vi "INI_DS1104Z.vi"(11 "VISA resource name":refnum<visa-resource-name>) -> (3 "VISA resource name out":refnum<visa-resource-name>)   [LabVIEW 2018]
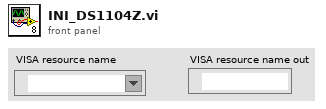
[diagram p1: front panel]
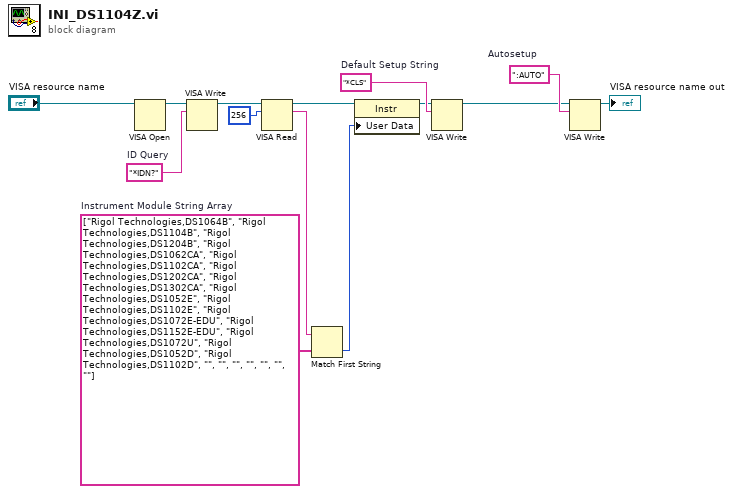
[diagram p0: block diagram]
diagram:
  w3 = ":AUTO"  # Autosetup
  w5 = "*CLS"  # Default Setup String
  w7 = string[] ["Rigol Technologies,DS1064B", "Rigol Technologies,DS1104B", "Rigol Technologies,DS1204B", "Rigol Technologies,DS1062CA", "Rigol Technologies,DS1102CA", "Rigol Technologies,DS1202CA", "Rigol Technologies,DS1302CA", "Rigol Technologies,DS1052E", "Rigol Technologies,DS1102E", "Rigol Technologies,DS1072E-EDU", "Rigol Technologies,DS1152E-EDU", "Rigol Technologies,DS1072U", "Rigol Technologies,DS1052D", "Rigol Technologies,DS1102D", "", "", "", "", "", "", ""]  # Instrument Module String Array
  w8 = "*IDN?"  # ID Query
  n1 = VISA Open(VISA resource name="VISA resource name") -> (VISA resource name=w11:refnum<visa-resource-name>)  [unwired: 1 in, 4 out]
  n2 = VISA Write(VISA resource name=w11, write buffer=w8) -> (VISA resource name out=w10:refnum<visa-resource-name>)  [unwired: 1 in, 2 out]
  n3 = VISA Read(VISA resource name=w10, byte count=u32 256) -> (VISA resource name out=w13:refnum<visa-resource-name>, read buffer=w6:string)  [unwired: 1 in, 2 out]
  n4 = Match First String(2:w7, 3:w6) -> (0:w12:i32)  [unwired: 1 out]
  n5 = property class="Instr"(reference=w13, "User Data"=w12) -> (reference out=w4:refnum<visa-resource-name>)  [unwired: 1 in, 1 out]
  n6 = VISA Write(VISA resource name=w4, write buffer=w5) -> (VISA resource name out=w2:refnum<visa-resource-name>)  [unwired: 1 in, 2 out]
  n7 = VISA Write(VISA resource name=w2, write buffer=w3) -> (VISA resource name out=→"VISA resource name out":refnum<visa-resource-name>)  [unwired: 1 in, 2 out]
